vi "3.vi"() -> ()   [LabVIEW 2020]
panel:
  in  "STOP":bool
  out "Overlimit?":bool
  in  "Limit [ms]":u32
  out "Counter [ms]":u32
  in  "Reset(T)/Count(F)":bool
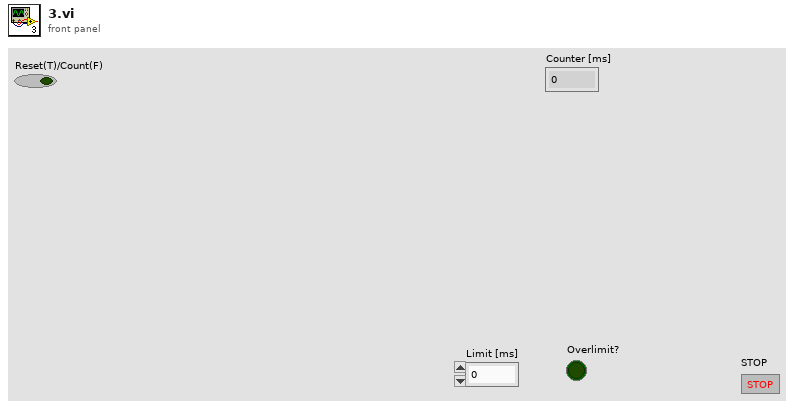
[diagram p1: front panel]
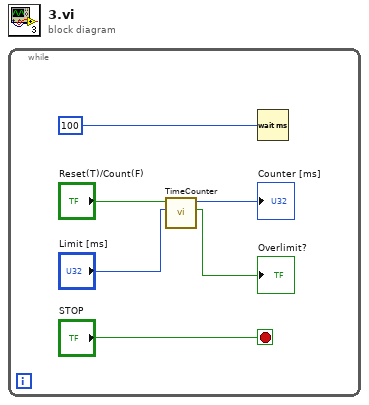
[diagram p0: block diagram]
diagram:
  n1 = while {
    stop <- "STOP" stop-if-true
    n2 = call "TimeCounter.vi"("Limit [ms]"="Limit [ms]", "Reset(T)/Count(F)"="Reset(T)/Count(F)") -> ("Overlimit?"=→"Overlimit?":bool, "Counter [ms]"=→"Counter [ms]":u32)  [unwired: 8 in]
    n3 = Wait (ms)(milliseconds to wait=u32 100) -> ()  [unwired: 1 out]
  }
